vi "OnShapeLV.vi"() -> ()   [LabVIEW 2019]
panel:
  in  "did":string
  in  "Name of the Document":string
  in  "rename document":bool
  in  "new document":bool
  out "Output Body":string
  out "Output headers":string
  in  "list document":bool
  # "do not need to enter\nname or did .. it will list\nall the documents \nregistered with the API"
  # "to rename a doc- enter the did and new name and click the button below"
  # "to create a new doc enter a name and click the button below"
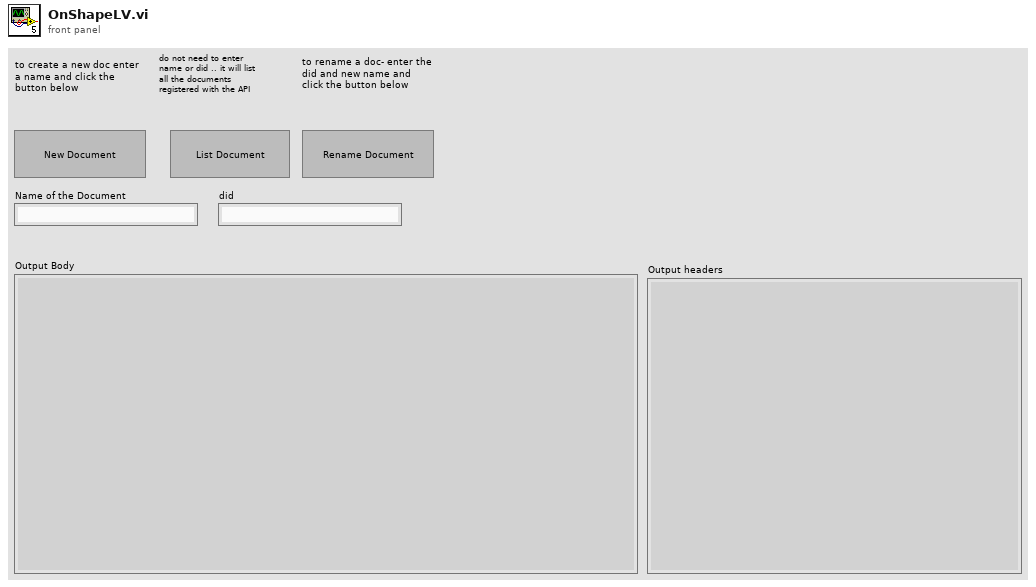
[diagram p1: front panel]
types:
  T1 = cluster{"name":string, "ownerType":i32, "isPublic":bool}
  T2 = cluster{"Date":string, "On-Nonce":string, "ctype":string, "path":string, "method":string, "Authorization":string, "Accept":string, "User-Agent":string, "Content-Type":string, "secret_key":string, "access_key":string, "stack":string, "payload":string}
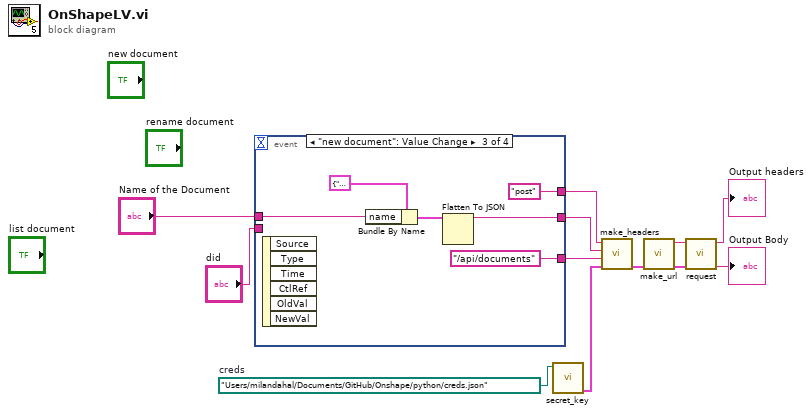
[diagram p0: block diagram]
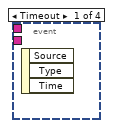
[diagram p2: hidden frame]
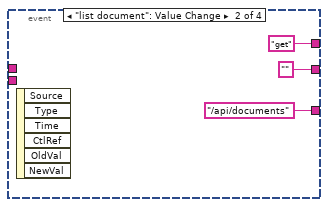
[diagram p3: hidden frame]
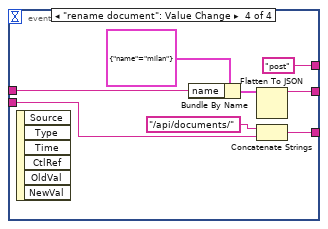
[diagram p4: hidden frame]
diagram:
  w12 = path "/Users/milandahal/Documents/GitHub/Onshape/python/creds.json"  # creds
  n1 = event shown="[2] \"new document\": Value Change" {
    selector: _ -> [_ _ _ _]
    dyn-events: _ -> [_ _ _ _]
    timeout: _ -> [_ _ _ _]
    tunnel: [_ "get" ("Method") "post" ("Method") "post" ("Method")] -> w7
    tunnel: [_ "" ("payload") w20 w26] -> w6
    tunnel: "Name of the Document" -> [_ _ w16 w25]
    tunnel: [_ "/api/documents" ("payload") "/api/documents" ("payload") w22] -> w2
    tunnel: "did" -> [_ _ _ w23]
    event Timeout {
      n2 = event-data() -> ()  [unwired: 1 in, 3 out]
    }
    event "list document": Value Change {
      n3 = event-data() -> ()  [unwired: 1 in, 6 out]
    }
    event "new document": Value Change {
      n4 = event-data() -> ()  [unwired: 1 in, 6 out]
      n5 = Bundle By Name(cluster=T1 {"name"="milan", "ownerType"=0, "isPublic"=FALSE}, "name"=w16) -> (w18:T1)
      n6 = Flatten To JSON(anything=w18) -> (JSON string=w20:string)  [unwired: 2 in, 1 out]
    }
    event "rename document": Value Change {
      n7 = event-data() -> ()  [unwired: 1 in, 6 out]
      n8 = Bundle By Name(cluster=cluster{"name":string} {"name"="milan"}, "name"=w25) -> (w28:cluster{"name":string})
      n9 = Flatten To JSON(anything=w28) -> (JSON string=w26:string)  [unwired: 2 in, 1 out]
      n10 = Concatenate Strings("/api/documents/" ("payload"), w23) -> (w22:string)
    }
  }
  n11 = call "secret_key.vi"("creds"=w12) -> ("output cluster"=w11:T2)  [unwired: 10 in]
  n12 = call "make_headers.vi"("Method"=w7, "payload"=w6, "path"=w2, "input"=w11) -> ("output cluster"=w8:T2)  [unwired: 5 in, 1 out]
  n13 = call "make_url.vi"("input cluster"=w8) -> ("Url"=w9:string, "input cluster 2"=w10:T2)  [unwired: 8 in]
  n14 = call "request.vi"("url"=w9, "input cluster"=w10) -> ("Output headers"=→"Output headers":string, "Output Body"=→"Output Body":string)  [unwired: 6 in]
